vi "DN4_SnapCounter_SetEventsToSnap.vi"(2 "events to snap":i32[](array[numeric]), 3 "error in (no error)":errorcluster, 4 "Task ID":u32) -> (0 "error out":errorcluster, 1 "Task ID out":u32)   [LabVIEW 2009]
uses:
  Windows/System32/AdvLvDaq.dll
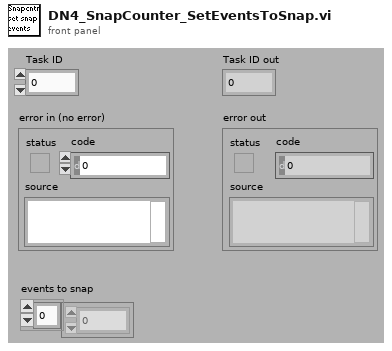
[diagram p1: front panel]
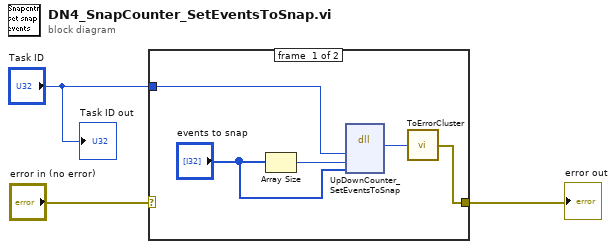
[diagram p0: block diagram]
diagram:
  n1 = case shown="No Error" "error in (no error)" {
    selector: "error in (no error)" -> [_ w9]
    tunnel: "Task ID" -> [w6 _]
    tunnel: [w4 w9] -> w2
    frame #0 {
      n2 = Array Size(array="events to snap") -> (size(s)=w8:i32)
      n3 = dll-call lib="C:/Windows/System32/AdvLvDaq.dll" fn="UpDownCounter_SetEventsToSnap"("taskID"=w6, "count"=w8, "events"="events to snap") -> ("return type"=w5:i32)  [unwired: 6 in, 2 out]
      n4 = call <userlib>:"ToErrorCluster.vi"("error code"=w5) -> ("error out"=w4:errorcluster)
    }
    frame #1 {
    }
  }
  "error out" <- w2
  "Task ID out" <- "Task ID"
